vi "CAN_Stop.vi"() -> ()   [LabVIEW 2020]
uses:
  Libraries/ZLG_CAN/ZLG_CAN.lvlib
panel:
  in  "索引":u32(ring) items=["0", "1", "2", "3", "4", "5", "6", "7", "8"]
  in  "设备类型":u32(ring)=27 items=["PCI5121"=1, "PCI9810"=2, "USBCAN1"=3, "USBCAN2"=4, "PCI9820"=5, "PCI5110"=7, "PC104CAN"=11, "CANETUDP"=12, "PCI9840B"=14, "PC104C2"=15, "PCI9820I"=16, "CANETTCP"=17, "PCIE9221"=24, "PCI5010U"=19, "USBCAN_E_U"=20, "USBCAN_2E_U"=21, "PCI5020U"=22, "PCIE9120I"=27, "PCIE9110I"=28, "PCIE9140I"=29]
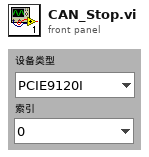
[diagram p1: front panel]
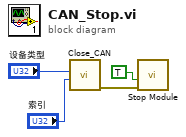
[diagram p0: block diagram]
diagram:
  n1 = call "Close_CAN.vi"("索引"="索引", "设备类型"="设备类型") -> ("error out"=w1:errorcluster)  [unwired: 9 in]
  n2 = call "Stop Module.vi"("error in (no error)"=w1, "Wait for Module to Stop? (F)"=TRUE) -> ()  [unwired: 9 in, 1 out]
